vi "write_basic_log.vi"(11 "NotifierReff":T1) -> (3 "xml string":string)   [LabVIEW 2013]
uses:
  cRIO_Code/Data/TypeDefs/Notifiers.ctl
  cRIO_Code/Data/TypeDefs/UTM Location.ctl
  cRIO_Code/Data/TypeDefs/Sail Set Suggestions.ctl
  cRIO_Code/Data/TypeDefs/Rudder Set Suggestions.ctl
  cRIO_Code/Data/TypeDefs/OverrideInformation.ctl
  cRIO_Code/Data/TypeDefs/OverrideMode.ctl
  cRIO_Code/Data/TypeDefs/MotorSetup.ctl
  cRIO_Code/Data/TypeDefs/DynamixelSetupInfo.ctl
  cRIO_Code/Data/TypeDefs/AirmarStatus.ctl
  cRIO_Code/Data/TypeDefs/HardwareOnline.ctl
  cRIO_Code/Data/TypeDefs/DynamixelCycleTracker.ctl
  cRIO_Code/Data/TypeDefs/RC Input Values.ctl
  cRIO_Code/Logic/Classes/Waypoint/Waypoint.lvclass
panel:
  out "Array":cluster{"name":string, "log value":string}[](array[cluster])
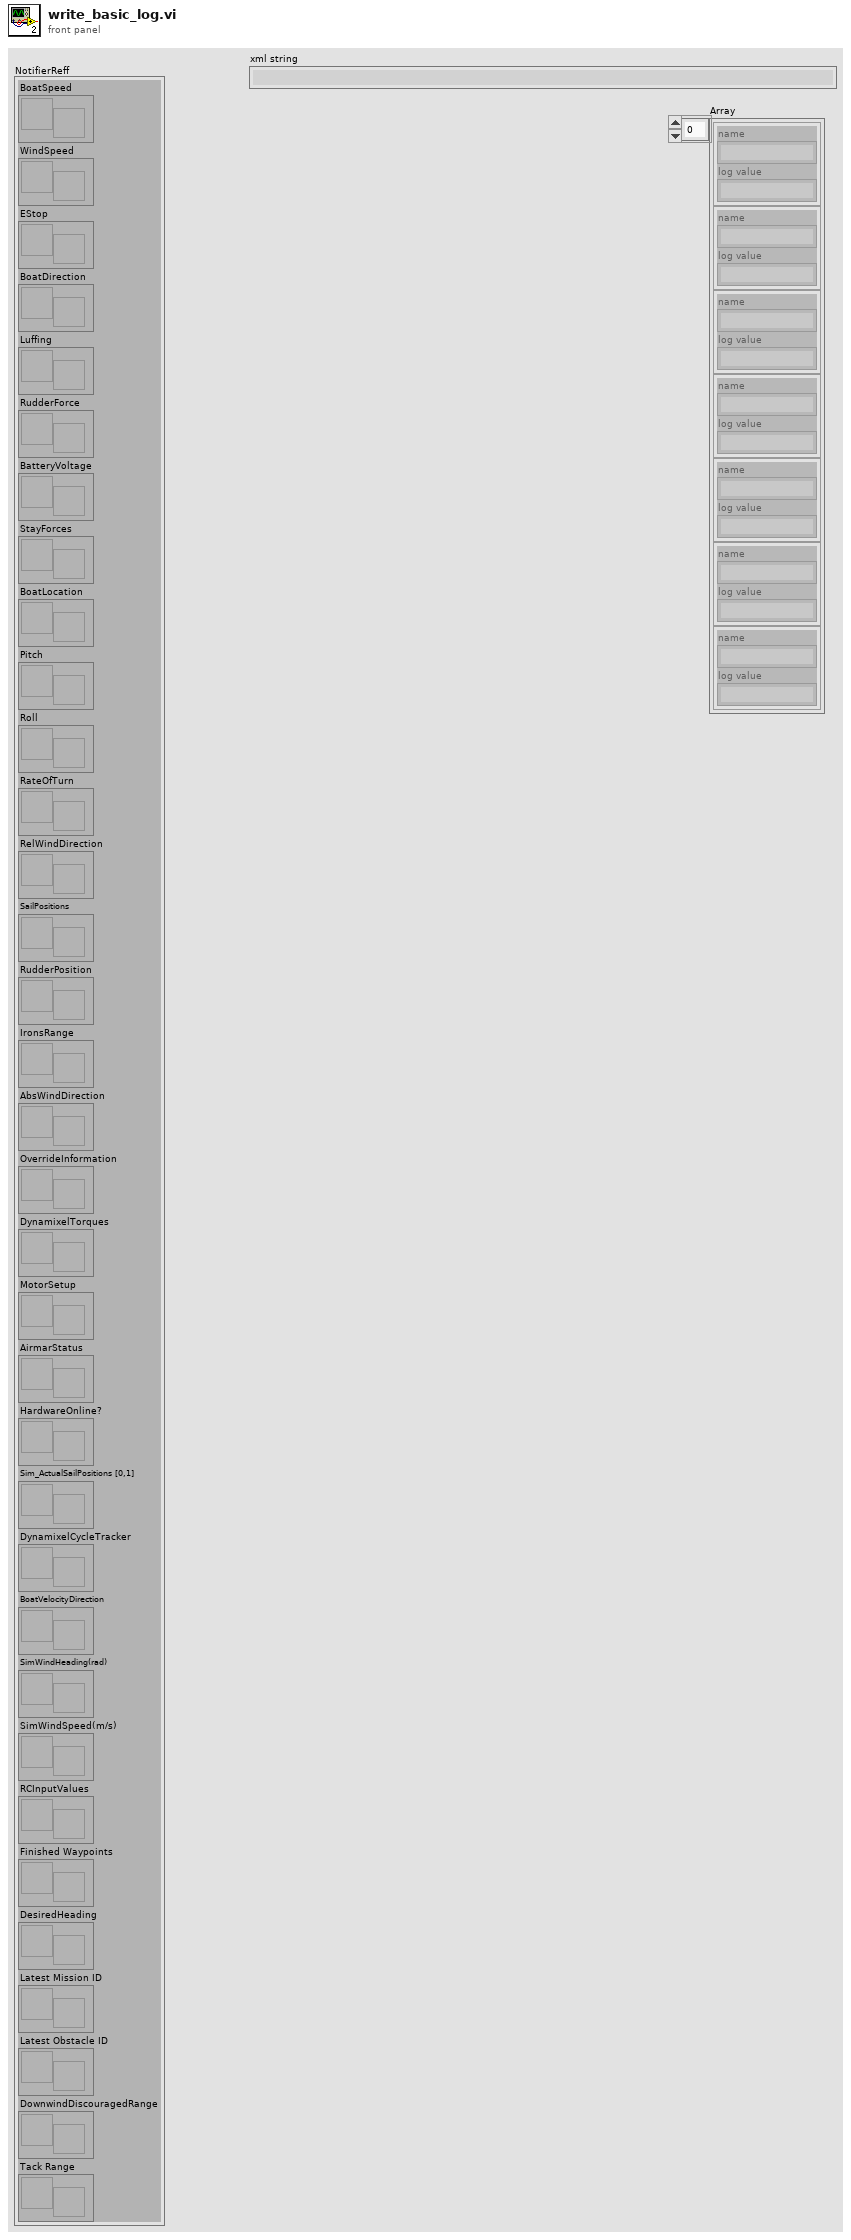
[diagram p1: front panel]
types:
  T1 = typedef "Notifiers.ctl" = cluster{"BoatSpeed":refnum<notifier>, "WindSpeed":refnum<notifier>, "EStop":refnum<notifier>, "BoatDirection":refnum<notifier>, "Luffing":refnum<notifier>, "RudderForce":refnum<notifier>, "BatteryVoltage":refnum<notifier>, "StayForces":refnum<notifier>, "BoatLocation":refnum<notifier>, "Pitch":refnum<notifier>, "Roll":refnum<notifier>, "RateOfTurn":refnum<notifier>, "RelWindDirection":refnum<notifier>, "SailPositions":refnum<notifier>, "RudderPosition":refnum<notifier>, "IronsRange":refnum<notifier>, "AbsWindDirection":refnum<notifier>, "OverrideInformation":refnum<notifier>, "DynamixelTorques":refnum<notifier>, "MotorSetup":refnum<notifier>, "AirmarStatus":refnum<notifier>, "HardwareOnline?":refnum<notifier>, "Sim_ActualSailPositions [0,1]":refnum<notifier>, "DynamixelCycleTracker":refnum<notifier>, "BoatVelocityDirection":refnum<notifier>, "SimWindHeading(rad)":refnum<notifier>, "SimWindSpeed(m/s)":refnum<notifier>, "RCInputValues":refnum<notifier>, "Finished Waypoints":refnum<notifier>, "DesiredHeading":refnum<notifier>, "Latest Mission ID":refnum<notifier>, "Latest Obstacle ID":refnum<notifier>, "DownwindDiscouragedRange":refnum<notifier>, "Tack Range":refnum<notifier>}
  T2 = typedef "Sail Set Suggestions.ctl" = cluster{"MainSailSuggestion":dbl, "JibSailSuggestion":dbl}
  T3 = typedef "Rudder Set Suggestions.ctl" = dbl
  T4 = typedef "UTM Location.ctl" = cluster{"UTM Zone":dbl, "Hemisphere":enum16{"North", "South"}, "East":dbl, "North":dbl}
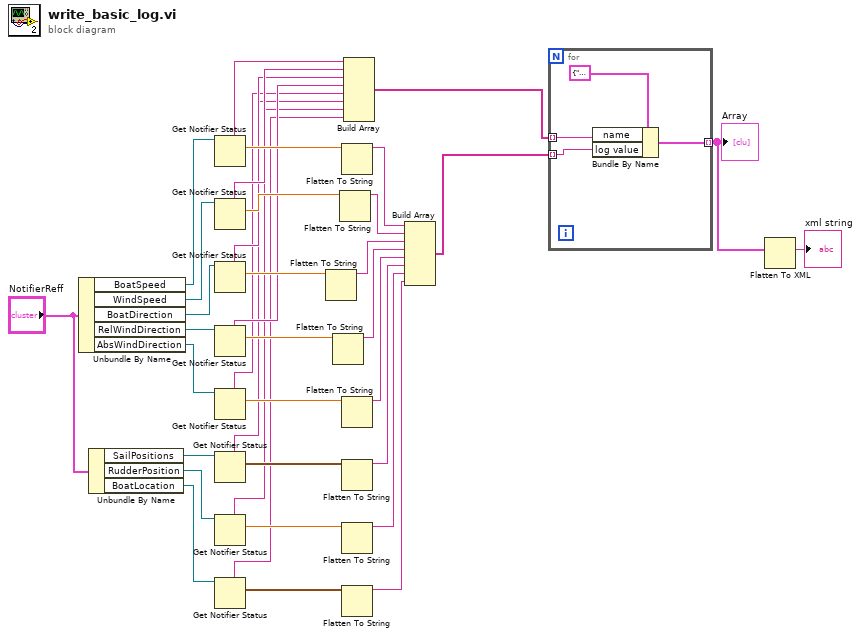
[diagram p0: block diagram]
diagram:
  n1 = Unbundle By Name("NotifierReff") -> ("BoatSpeed"=w27:refnum<notifier>, "WindSpeed"=w26:refnum<notifier>, "BoatDirection"=w25:refnum<notifier>, "RelWindDirection"=w24:refnum<notifier>, "AbsWindDirection"=w23:refnum<notifier>)
  n2 = Unbundle By Name("NotifierReff") -> ("SailPositions"=w36:refnum<notifier>, "RudderPosition"=w35:refnum<notifier>, "BoatLocation"=w34:refnum<notifier>)
  n3 = Get Notifier Status(notifier=w27) -> (notifier name=w17:string, current notification=w22:dbl)  [unwired: 1 in, 3 out]
  n4 = Get Notifier Status(notifier=w26) -> (notifier name=w16:string, current notification=w21:dbl)  [unwired: 1 in, 3 out]
  n5 = Get Notifier Status(notifier=w25) -> (notifier name=w15:string, current notification=w20:dbl)  [unwired: 1 in, 3 out]
  n6 = Get Notifier Status(notifier=w24) -> (notifier name=w14:string, current notification=w19:dbl)  [unwired: 1 in, 3 out]
  n7 = Get Notifier Status(notifier=w23) -> (notifier name=w13:string, current notification=w18:dbl)  [unwired: 1 in, 3 out]
  n8 = Get Notifier Status(notifier=w36) -> (notifier name=w12:string, current notification=w31:T2)  [unwired: 1 in, 3 out]
  n9 = Get Notifier Status(notifier=w35) -> (notifier name=w11:string, current notification=w32:T3)  [unwired: 1 in, 3 out]
  n10 = Get Notifier Status(notifier=w34) -> (notifier name=w10:string, current notification=w33:T4)  [unwired: 1 in, 3 out]
  n11 = Flatten To String(anything=w20) -> (data string=w7:string)  [unwired: 3 in, 2 out]
  n12 = Flatten To String(anything=w19) -> (data string=w8:string)  [unwired: 3 in, 2 out]
  n13 = Flatten To String(anything=w21) -> (data string=w6:string)  [unwired: 3 in, 2 out]
  n14 = Flatten To String(anything=w22) -> (data string=w5:string)  [unwired: 3 in, 2 out]
  n15 = Flatten To String(anything=w18) -> (data string=w9:string)  [unwired: 3 in, 2 out]
  n16 = Flatten To String(anything=w31) -> (data string=w30:string)  [unwired: 3 in, 2 out]
  n17 = Flatten To String(anything=w32) -> (data string=w29:string)  [unwired: 3 in, 2 out]
  n18 = Flatten To String(anything=w33) -> (data string=w28:string)  [unwired: 3 in, 2 out]
  n19 = Build Array(w17, w16, w15, w14, w13, w12, w11, w10) -> (w4:string[])
  n20 = Build Array(w5, w6, w7, w8, w9, w30, w29, w28) -> (w3:string[])
  n21 = for {
    tunnel: w4 -> [w40] mode=indexing
    tunnel: w3 -> [w39] mode=indexing
    tunnel: [w38] -> w2 mode=indexing
    n22 = Bundle By Name(cluster=cluster{"name":string, "log value":string} {"name"="", "log value"=""}, "name"=w40, "log value"=w39) -> (w38:cluster{"name":string, "log value":string})
  }
  "Array" <- w2
  n23 = Flatten To XML(anything=w2) -> (xml string=→"xml string":string)
